vi "ReadText_StepbyStep.vi"() -> ()   [LabVIEW 2018]
panel:
  in  "Activate Time":dbl=5.0
  in  "stop":bool
  out "Index":i32=7
  out "element":string="50"
  out "X, Y, Z, S":i32=3
  out "size(s)":i32=8
  out "EOF?":bool
  in  "delimiter (Tab)":string="\t"
  in  "type (empty)":string[][](array[string])
  in  "transpose (no:F)":bool
  in  "format (%.3f)":string="%.3f"
  out "all rows":string[][](array[string])=[["10"], ["20"], ["30"], ["0"], ["40"], ["50"], ["60"], ["50"]]
  in  "number of rows (all:-1)":i32=-1
  out "mark after read (chars.)":i32=29
  in  "max characters/row  (no limit:0)":i32
  in  "start of read offset (chars.:0)":i32
  in  "file path (dialog if empty)":path=path "C:/Users/Academia Sinica/Desktop/AutoSampler _GB/AutoSampler.txt"
  # "(S)"
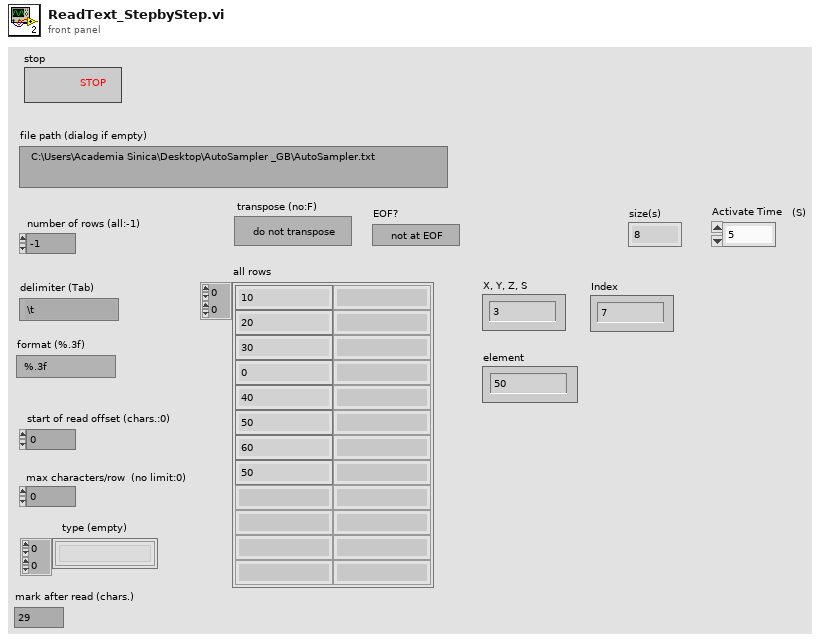
[diagram p1: front panel]
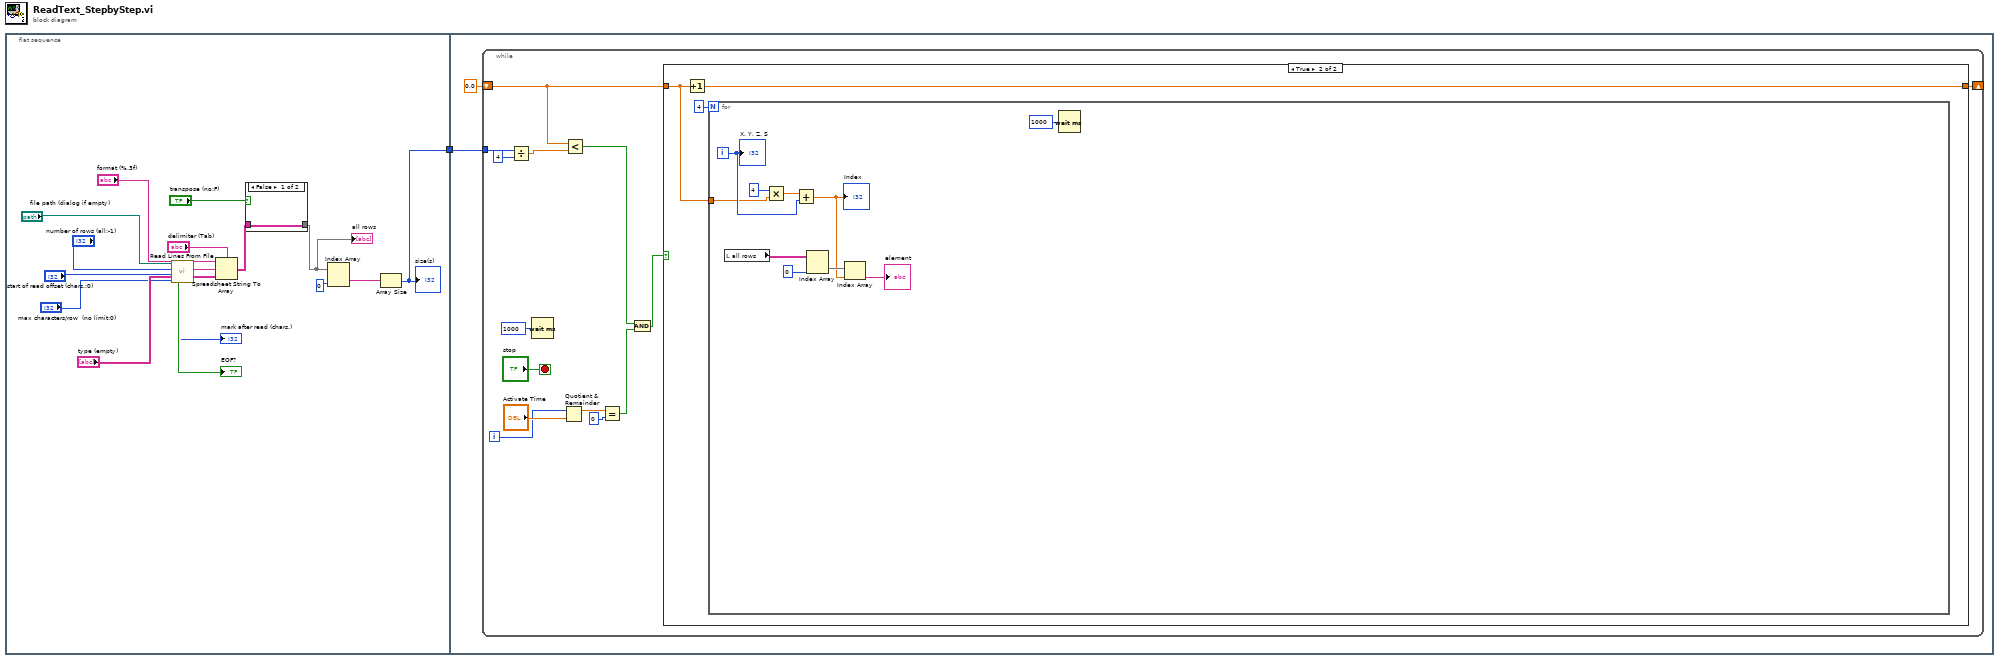
[diagram p0: block diagram]
diagram:
  n1 = flat-sequence {
    tunnel: [w2] -> w1
    tunnel: w1 -> [w21]
    frame #0 {
      n2 = call <vilib>:"Read Lines From File.vi"("file path (dialog if empty)"="file path (dialog if empty)", "number of lines (all:-1)"="number of rows (all:-1)", "start of read offset (chars.:0)"="start of read offset (chars.:0)", "[max characters per line]  (no limit:0)"="max characters/row  (no limit:0)") -> ("line string"=w9:string, "mark after read (chars.)"=→"mark after read (chars.)":i32, "EOF?"=→"EOF?":bool)  [unwired: 2 in, 1 out]
      n3 = Spreadsheet String To Array(delimiter (Tab)="delimiter (Tab)", format string="format (%.3f)", spreadsheet string=w9, array type (2D Dbl)="type (empty)") -> (array=w11:string[][])
      n4 = case shown="False" "transpose (no:F)" {
        tunnel: [w18 w20] -> w17
        tunnel: w11 -> [w18 w19]
        frame False {
        }
        frame True {
          n5 = Transpose 2D Array(2D array=w19) -> (transposed array=w20:string[][])
        }
      }
      "all rows" <- w17
      n6 = Index Array "Index Array"(array=w17, index (col)=0) -> (element=w3:string[])  [unwired: 1 in]
      n7 = Array Size(array=w3) -> (size(s)=w2:i32)
      "size(s)" <- w2
    }
    frame #1 {
      n8 = while {
        shift-right: [w30] -> _
        shift-left: 0.0 ("Numeric") -> [w28]
        tunnel: w21 -> [w25]
        i -> [w32]
        stop <- "stop" stop-if-true
        n9 = Divide(x=w25, y=4) -> (x/y=w23:dbl)
        n10 = Wait (ms)(milliseconds to wait=u32 1000) -> ()  [unwired: 1 out]
        n11 = Quotient & Remainder(x=w32, y="Activate Time") -> (x-y*floor(x/y)=w35:dbl)  [unwired: 1 out]
        n12 = Less?(x=w28, y=w23) -> (x < y?=w27:bool)
        n13 = Equal?(x=w35, y=0) -> (x = y?=w29:bool)
        n14 = And(x=w27, y=w29) -> (x .and. y?=w26:bool)
        n15 = case shown="True" w26 {
          tunnel: w28 -> [w37 w38]
          tunnel: [w37 w39] -> w30
          frame False {
          }
          frame True {
            n16 = Increment(x=w38) -> (x+1=w39:dbl)
            n17 = for {
              N: 4 -> [_]
              tunnel: w38 -> [w42]
              i -> [w48]
              n18 = local read "all rows"() -> (w47:string[][])
              n19 = Multiply(x=4, y=w42) -> (x*y=w50:dbl)
              n20 = Add(x=w50, y=w48) -> (x+y=w44:dbl)
              "Index" <- w44
              n21 = Index Array "Index Array"(array=w47, index (col)=0 ("disabled index (col)")) -> (element=w45:string[])  [unwired: 1 in]
              n22 = Index Array(array=w45, index=w44) -> (element=→"element":string)
              n23 = Wait (ms)(milliseconds to wait=u32 1000) -> ()  [unwired: 1 out]
              "X, Y, Z, S" <- w48
            }
          }
        }
      }
    }
  }
